vi "Check Message Queue Status.vi"(7 "error in (no error)":errorcluster, 10 "Message queue in":T1) -> (0 "error out":errorcluster, 2 "# elements in queue":i32, 3 "Message queue out":T1)   [LabVIEW 2014, in "AMC.lvlib"]
uses:
  AMC.lvlib
  _SubVIs/TypeDefs/Message Queue.ctl
  _SubVIs/TypeDefs/Message.ctl
  Keyed Array/KeyedArray.ctl
  Keyed Array/Tools_KeyedArray.lvlib
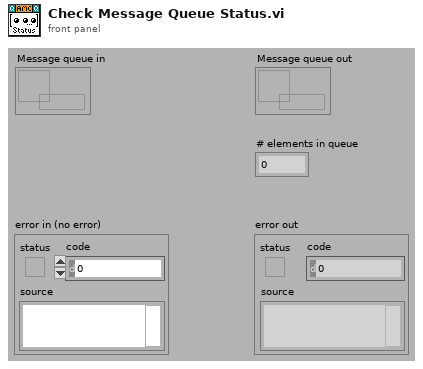
[diagram p1: front panel]
types:
  T1 = typedef "AMC.lvlib/Message Queue.ctl" = refnum<queue>
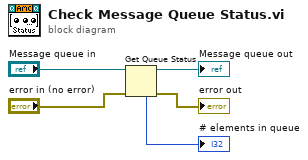
[diagram p0: block diagram]
diagram:
  n1 = Get Queue Status(queue="Message queue in", error in (no error)="error in (no error)") -> (queue out=→"Message queue out":T1, error out=→"error out":errorcluster, # elements in queue=→"# elements in queue":i32)  [unwired: 6 out]
